vi "Save Signal Config.vi"(8 "error in":errorcluster, 10 "SignalConfig":T1) -> (0 "error out":errorcluster)   [LabVIEW 2020, in "DataBase.lvlib"]
doc: "_____\nCreated using Delacor QMH Event Scripter 6.0.0.121."
uses:
  DataBase.lvlib
  Acquisition/SignalConfig--cluster.ctl
  Save Signal Config Argument--cluster.ctl
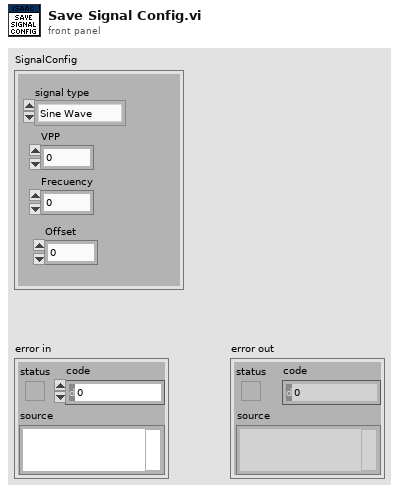
[diagram p1: front panel]
types:
  T1 = typedef "SignalConfig--cluster.ctl" = cluster{"VPP":i32, "Frecuency":dbl, "Offset":dbl, "signal type":enum16{"Sine Wave", "Triangle Wave", "Square Wave", "Sawtooth Wave"}}
  T2 = typedef "DataBase.lvlib/Save Signal Config Argument--cluster.ctl" = cluster{"SignalConfig":T1}
  T3 = typedef "DataBase.lvlib/Request Events--cluster.ctl" = cluster{"Stop Module":refnum<user-event>, "Show Panel":refnum<user-event>, "Hide Panel":refnum<user-event>, "Get Module Execution Status":refnum<user-event>, "Show Diagram":refnum<user-event>, "Fetch Data":refnum<user-event>, "Save config":refnum<user-event>, "Save Signal Config":refnum<user-event>}
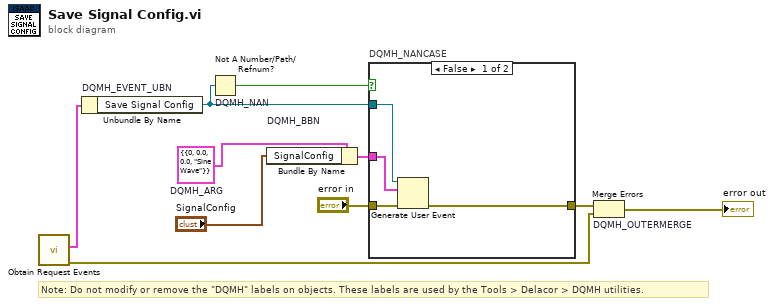
[diagram p0: block diagram]
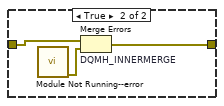
[diagram p2: hidden frame]
diagram:
  w4 = T2 {"SignalConfig"={"VPP"=0, "Frecuency"=0.0, "Offset"=0.0, "signal type"=enum."Sine Wave"}}  # DQMH_ARG
  # "Note: Do not modify or remove the \"DQMH\" labels on objects. These labels are used by the Tools > Delacor > DQMH utilities."
  n1 = call "Obtain Request Events.vi"() -> ("error out"=w2:errorcluster, "DataBase Request Events"=w1:T3)  [unwired: 10 in]
  n2 = Unbundle By Name "DQMH_EVENT_UBN"(w1) -> ("Save Signal Config"=w6:refnum<user-event>)
  n3 = Not A Number/Path/Refnum? "DQMH_NAN"(number/path/refnum=w6) -> (NaN/Path/Refnum?=w7:bool)
  n4 = Bundle By Name "DQMH_BBN"(cluster=w4, "SignalConfig"="SignalConfig") -> (w8:T2)
  n5 = case "DQMH_NANCASE" shown="False" w7 {
    tunnel: "error in" -> [w14 w17]
    tunnel: [w13 w16] -> w5
    tunnel: w6 -> [w12 _]
    tunnel: w8 -> [w11 _]
    frame False {
      n6 = Generate User Event(user event=w12, event data cluster=w11, error in=w14) -> (error out=w13:errorcluster)  [unwired: 1 in, 1 out]
    }
    frame True {
      n7 = call "Module Not Running--error.vi"() -> ("error out"=w15:errorcluster)  [unwired: 11 in]
      n8 = Merge Errors "DQMH_INNERMERGE"(w17, w15) -> (w16:errorcluster)
    }
  }
  n9 = Merge Errors "DQMH_OUTERMERGE"(w5, w2) -> (→"error out":errorcluster)
